vi "Longest common subsequence.vi"(9 "Pattern 2 COLUMN(0)":string="0 1 -4 4 -4 0 -3 3 0 -2 3", 11 "Pattern 1 ROW(0)":string="0 -1 0 4 -3 0 2 -2 3") -> (1 "LCS length":dbl, 3 "LCS array":dbl[][](array[numeric]))   [LabVIEW 2014]
panel:
  out "innitial array":dbl[][](array[numeric])
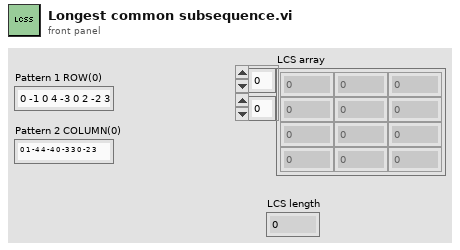
[diagram p1: front panel]
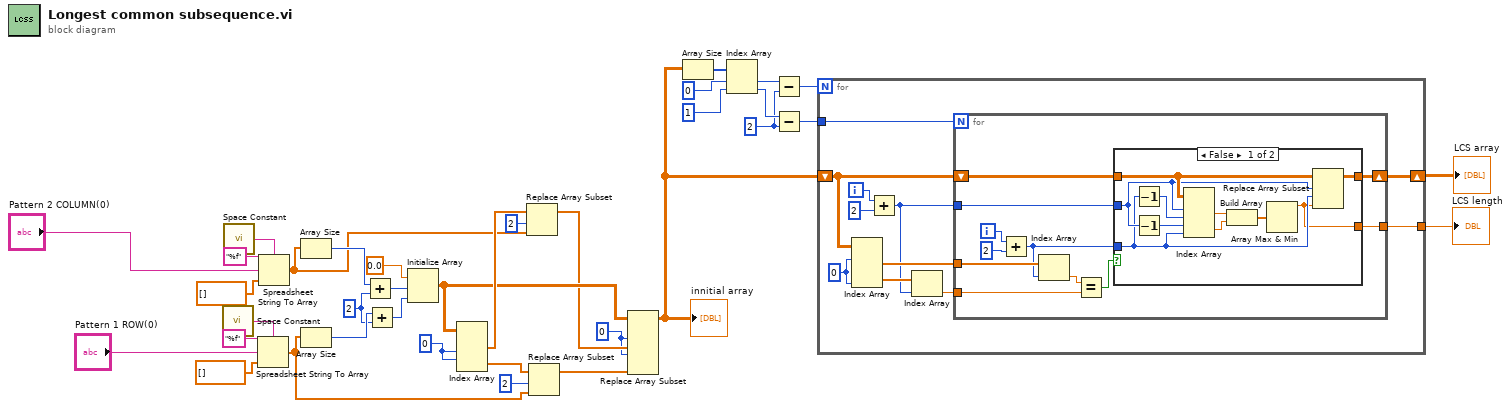
[diagram p0: block diagram]
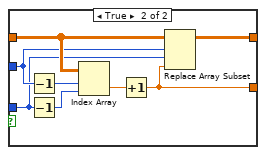
[diagram p2: hidden frame]
diagram:
  w5 = 2 ("y")
  w2 = 0 ("index (row)")
  w3 = 0 ("index (row)")
  w25 = 2 ("y")
  n1 = call <vilib>:"Space Constant.vi"() -> ("String"=w32:string)
  n2 = call <vilib>:"Space Constant.vi"() -> ("String"=w35:string)
  n3 = Spreadsheet String To Array(delimiter (Tab)=w32, format string="%f", spreadsheet string="Pattern 1 ROW(0)", array type (2D Dbl)=dbl[] [] ("array 2")) -> (array=w19:dbl[])
  n4 = Spreadsheet String To Array(delimiter (Tab)=w35, format string="%f", spreadsheet string="Pattern 2 COLUMN(0)", array type (2D Dbl)=dbl[] [] ("array 2")) -> (array=w23:dbl[])
  n5 = Array Size(array=w23) -> (size(s)=w27:i32)
  n6 = Array Size(array=w19) -> (size(s)=w26:i32)
  n7 = Add(x=w27, y=w25) -> (x+y=w30:i32)
  n8 = Add(x=w26, y=w25) -> (x+y=w29:i32)
  n9 = Initialize Array(0.0, w30, w29) -> (w18:dbl[][])
  n10 = Index Array(array=w18, index (col) #1=w3, index (row) #2=w3) -> (element #1=w24:dbl[], element #2=w20:dbl[])  [unwired: 2 in]
  n11 = Replace Array Subset(array=w24, new element=w23, index=2) -> (w17:dbl[])
  n12 = Replace Array Subset(array=w20, new element=w19, index=2) -> (w16:dbl[])
  n13 = Replace Array Subset(array=w18, new element #1=w17, index (col) #1=w2, new element #2=w16, index (row) #2=w2) -> (w15:dbl[][])  [unwired: 2 in]
  "innitial array" <- w15
  n14 = Array Size(array=w15) -> (size(s)=w14:i32[])
  n15 = Index Array(array=w14, index #1=0 ("index"), index #2=1 ("index")) -> (element #1=w11:i32, element #2=w6:i32)
  n16 = Subtract(x=w11, y=w5) -> (x-y=w12:i32)
  n17 = Subtract(x=w6, y=w5) -> (x-y=w4:i32)
  n18 = for {
    N: w12 -> [_]
    shift-right: [w45] -> w10
    shift-left: w15 -> [w46]
    tunnel: w4 -> [w44]
    tunnel: [w37] -> w1
    i -> [w41]
    w47 = 0 ("index (row)")
    n19 = Index Array(array=w46, index (row) #1=w47, index (col) #2=w47) -> (element #1=w39:dbl[], element #2=w42:dbl[])  [unwired: 2 in]
    n20 = Add(x=w41, y=2) -> (x+y=w38:i32)
    n21 = Index Array(array=w42, index=w38) -> (element=w40:dbl)
    n22 = for {
      N: w44 -> [_]
      shift-right: [w49] -> w45
      shift-left: w46 -> [w52]
      tunnel: w40 -> [w54]
      tunnel: w39 -> [w57]
      tunnel: w38 -> [w51]
      tunnel: [w48] -> w37
      i -> [w56]
      n23 = Add(x=w56, y=2) -> (x+y=w50:i32)
      n24 = Index Array(array=w57, index=w50) -> (element=w55:dbl)
      n25 = Equal?(x=w55, y=w54) -> (x = y?=w53:bool)
      n26 = case shown="False" w53 {
        tunnel: w52 -> [w63 w75]
        tunnel: w51 -> [w62 w71]
        tunnel: w50 -> [w61 w70]
        tunnel: [w60 w72] -> w49
        tunnel: [w59 w69] -> w48
        frame False {
          n27 = Decrement(x=w61) -> (x-1=w68:i32)
          n28 = Decrement(x=w62) -> (x-1=w67:i32)
          n29 = Index Array(array=w63, index (row) #1=w62, index (col) #1=w68, index (row) #2=w67, index (col) #2=w61) -> (element #1=w66:dbl, element #2=w65:dbl)
          n30 = Build Array(w66, w65) -> (w64:dbl[])
          n31 = Array Max & Min(array=w64) -> (max value=w59:dbl)  [unwired: 3 out]
          n32 = Replace Array Subset(array=w63, new element=w59, index (row)=w62, index (col)=w61) -> (w60:dbl[][])
        }
        frame True {
          n33 = Decrement(x=w71) -> (x-1=w74:i32)
          n34 = Decrement(x=w70) -> (x-1=w73:i32)
          n35 = Index Array(array=w75, index (row)=w74, index (col)=w73) -> (element=w76:dbl)
          n36 = Increment(x=w76) -> (x+1=w69:dbl)
          n37 = Replace Array Subset(array=w75, new element=w69, index (row)=w71, index (col)=w70) -> (w72:dbl[][])
        }
      }
    }
  }
  "LCS array" <- w10
  "LCS length" <- w1
